vi "S1500_S7Com_BITtoBYTE.vi"(5 "Variant":variant, 7 "Cluster":T1={"DB"=0, "Adresse"=0, "Länge"=0, "Typ"=enum."BYTE", "Enum"=enum."WRITE"}, 8 "error in":errorcluster caption="Fehler (Eingang, kein Fehler)", 10 "RW Data":i32[](array[numeric])) -> (0 "error out":errorcluster caption="Fehler (Ausgang)", 2 "RW Data":i32[](array[numeric]))   [LabVIEW 2018]
uses:
  S1500_ENUM Typ.ctl
  S1500_S7Com_DATATypes.ctl
  S1500_S7Com_RW.ctl
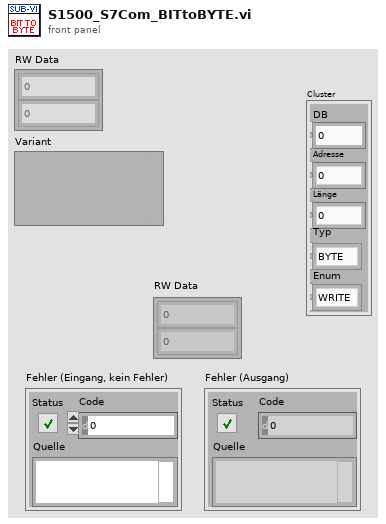
[diagram p1: front panel]
types:
  T1 = typedef "S1500_ENUM Typ.ctl" = cluster{"DB":u32, "Adresse":u32, "Länge":u32, "Typ":T2, "Enum":T3}
  T2 = typedef "S1500_S7Com_DATATypes.ctl" = enum16{"", "BIT", "BYTE", "CHAR", "WORD", "INT", "DWORD", "DINT", "REAL", "STRING"}
  T3 = typedef "S1500_S7Com_RW.ctl" = enum16{"WRITE", "READ"}
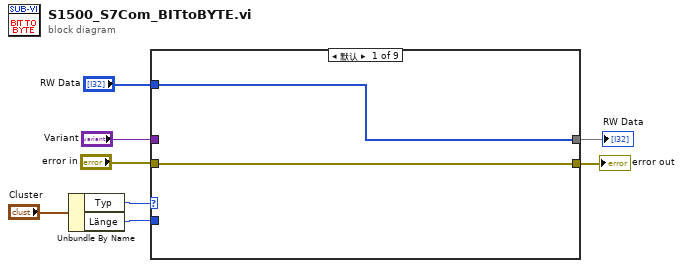
[diagram p0: block diagram]
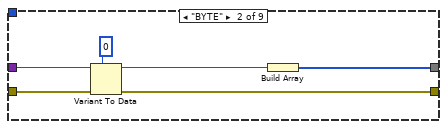
[diagram p2: hidden frame]
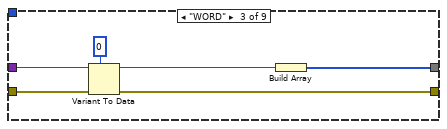
[diagram p3: hidden frame]
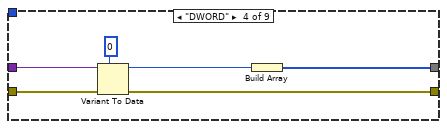
[diagram p4: hidden frame]
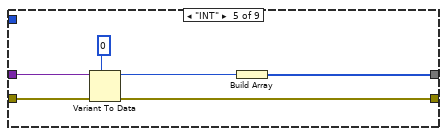
[diagram p5: hidden frame]
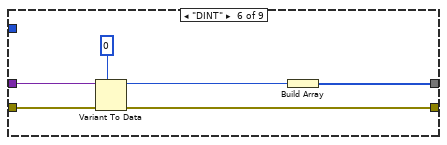
[diagram p6: hidden frame]
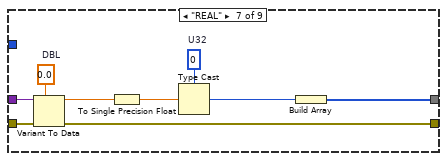
[diagram p7: hidden frame]
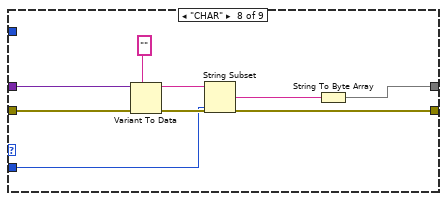
[diagram p8: hidden frame]
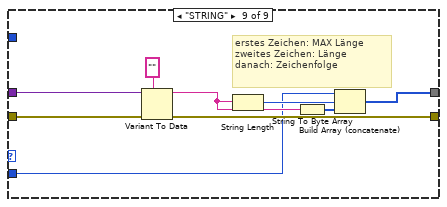
[diagram p9: hidden frame]
diagram:
  n1 = Unbundle By Name("Cluster") -> ("Typ"=w6:T2, "Länge"=w1:u32)
  n2 = case shown="默认" w6 {
    tunnel: [w10 w16 w22 w28 w31 w38 w41 w53 w58] -> w7
    tunnel: "Variant" -> [_ w15 w20 w25 w34 w39 w43 w57 w60]
    tunnel: "RW Data" -> [w10 _ _ _ _ _ _ _ _]
    tunnel: w1 -> [_ _ _ _ _ _ _ w52 w59]
    tunnel: "error in" -> [w9 w12 w18 w24 w30 w36 w44 w55 w61]
    tunnel: [w9 w11 w17 w23 w29 w35 w42 w54 w62] -> w2
    frame Default {
    }
    frame "BYTE" {
      n3 = Variant To Data(error in=w12, type=u8 0, Variant=w15) -> (data=w13:u8, error out=w11:errorcluster)
      n4 = Build Array(w13) -> (w16:u8[])
    }
    frame "WORD" {
      n5 = Variant To Data(error in=w18, type=u16 0, Variant=w20) -> (data=w19:u16, error out=w17:errorcluster)
      n6 = Build Array(w19) -> (w22:u16[])
    }
    frame "DWORD" {
      n7 = Variant To Data(error in=w24, type=u32 0, Variant=w25) -> (data=w26:u32, error out=w23:errorcluster)
      n8 = Build Array(w26) -> (w28:u32[])
    }
    frame "INT" {
      n9 = Variant To Data(error in=w30, type=i16 0, Variant=w34) -> (data=w32:i16, error out=w29:errorcluster)
      n10 = Build Array(w32) -> (w31:i16[])
    }
    frame "DINT" {
      n11 = Variant To Data(error in=w36, type=i16 0, Variant=w39) -> (data=w37:i16, error out=w35:errorcluster)
      n12 = Build Array(w37) -> (w38:i16[])
    }
    frame "REAL" {
      w46 = u32 0  # U32
      w45 = 0.0  # DBL
      n13 = Variant To Data(error in=w44, type=w45, Variant=w43) -> (data=w48:dbl, error out=w42:errorcluster)
      n14 = To Single Precision Float(number=w48) -> (single precision float=w47:sgl)
      n15 = Type Cast(type=w46, x=w47) -> (*(type *) &x=w49:u32)
      n16 = Build Array(w49) -> (w41:u32[])
    }
    frame "CHAR" {
      n17 = Variant To Data(error in=w55, type="", Variant=w57) -> (data=w51:string, error out=w54:errorcluster)
      n18 = String Subset(string=w51, length (rest)=w52) -> (substring=w50:string)  [unwired: 1 in]
      n19 = String To Byte Array(string=w50) -> (unsigned byte array=w53:u8[])
    }
    frame "STRING" {
      # "erstes Zeichen: MAX Länge\nzweites Zeichen: Länge\ndanach: Zeichenfolge"
      n20 = Variant To Data(error in=w61, type="", Variant=w60) -> (data=w63:string, error out=w62:errorcluster)
      n21 = String Length(string=w63) -> (length=w65:i32)
      n22 = String To Byte Array(string=w63) -> (unsigned byte array=w64:u8[])
      n23 = Build Array (concatenate)(w59, w65, w64) -> (w58:u32[])
    }
  }
  "RW Data" <- w7
  "error out" <- w2
